vi "Utility_Read_Mixture_Cluster.vi"(6 "error in (no error)":errorcluster, 8 "Dir containing fluid files":path, 9 "Mixture File":path) -> (0 "error out":errorcluster, 3 "Mixure Cluster":T1)   [LabVIEW 2015]
doc: "Reads the .mix file from the disk and retruns a cluster specifying the composition of the fluid.\n\nDeveloped by:\nGreg Sussman\nProcess Automation Corp\nwww.processauto.com\n(267)685-1249"
uses:
  Ctl/Mixture Composition cluster_d.ctl
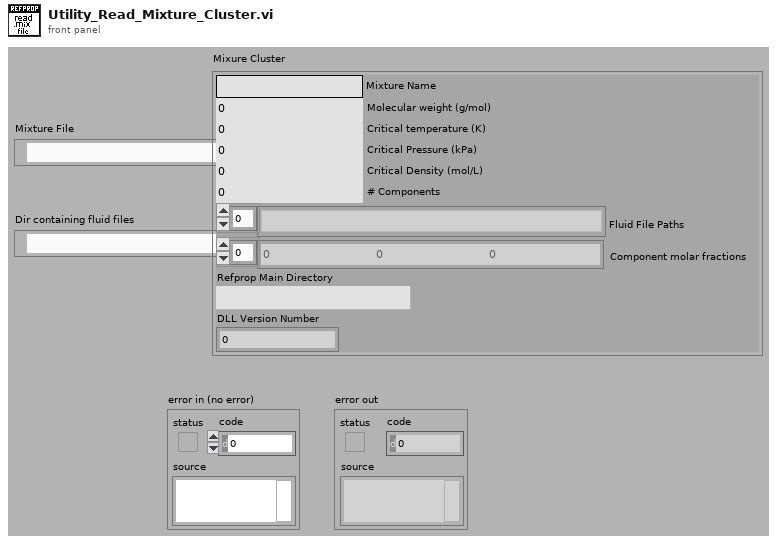
[diagram p1: front panel]
types:
  T1 = typedef "Mixture Composition cluster_d.ctl" = cluster{"Mixture Name":string, "Molecular weight (g/mol)":dbl, "Critical temperature (K)":dbl, "Critical Pressure (kPa)":dbl, "Critical Density (mol/L)":dbl, "# Components":i32, "Fluid File Paths":path[], "Component molar fractions":dbl[], "Refprop Main Directory":path, "DLL Version Number":dbl}
  T2 = enum16{"open", "open or create", "create or replace", "create", "open (read only)"}
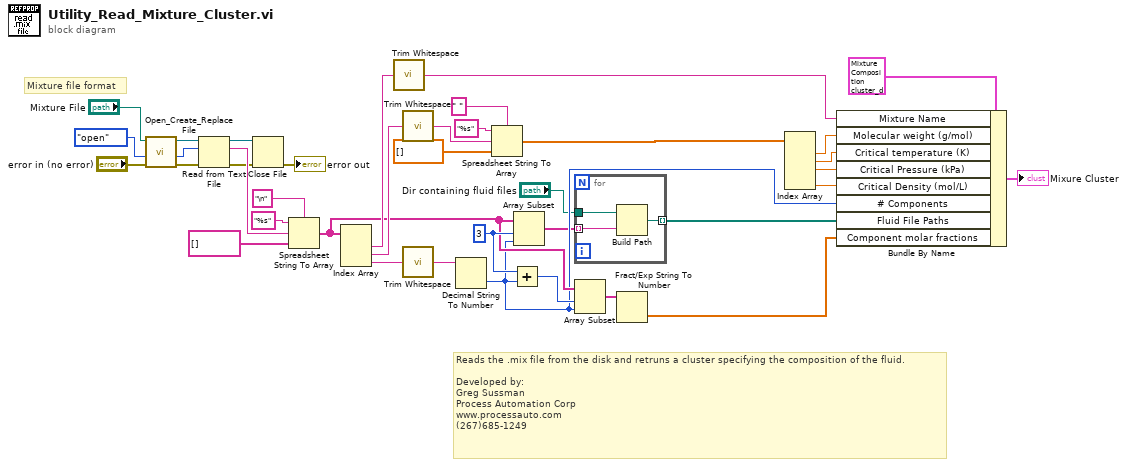
[diagram p0: block diagram]
diagram:
  w34 = 3 ("index")
  # "Reads the .mix file from the disk and retruns a cluster specifying the composition of the fluid.\n\nDeveloped by:\nGreg Sussman\nProcess Automation Corp\nwww.processauto.com\n(267)685-1249"
  # "Mixture file format"
  n1 = call <vilib>:"Open_Create_Replace File.vi"("error in (no error)"="error in (no error)", "function (open:0)"=T2."open", "file path"="Mixture File") -> ("error out"=w5:errorcluster, "file size (bytes)"=w1:i32, "refnum"=w4:refnum<file>)  [unwired: 5 in, 1 out]
  n2 = Read from Text File(file (use dialog)=w4, count=w1, error in=w5) -> (refnum out=w2:refnum<file>, text=w10:string, error out=w3:errorcluster)  [unwired: 1 in, 1 out]
  n3 = Close File(refnum=w2, error in=w3) -> (error out=→"error out":errorcluster)  [unwired: 1 out]
  n4 = Spreadsheet String To Array(delimiter (Tab)="\n", format string="%s", spreadsheet string=w10, array type (2D Dbl)=string[] []) -> (array=w18:string[])
  n5 = Index Array(array=w18) -> (element #1=w31:string, element #2=w24:string, element #3=w19:string)  [unwired: 3 in]
  n6 = call <vilib>:"Trim Whitespace.vi"("string"=w31) -> ("trimmed string"=w25:string)  [unwired: 1 in]
  n7 = call <vilib>:"Trim Whitespace.vi"("string"=w24) -> ("trimmed string"=w30:string)  [unwired: 1 in]
  n8 = call <vilib>:"Trim Whitespace.vi"("string"=w19) -> ("trimmed string"=w35:string)  [unwired: 1 in]
  n9 = Decimal String To Number(string=w35) -> (number=w17:i32)  [unwired: 2 in, 1 out]
  n10 = Spreadsheet String To Array(delimiter (Tab)=" ", format string="%s", spreadsheet string=w30, array type (2D Dbl)=dbl[] []) -> (array=w29:dbl[])
  n11 = Add(x=w34, y=w17) -> (x+y=w33:i32)
  n12 = Array Subset(array=w18, index=w34, length=w17) -> (w13:string[])
  n13 = for {
    tunnel: w13 -> [w41] mode=indexing
    tunnel: "Dir containing fluid files" -> [w40]
    tunnel: [w39] -> w11 mode=indexing
    n14 = Build Path(base path=w40, name or relative path=w41) -> (appended path=w39:path)
  }
  n15 = Array Subset(array=w18, index=w33, length=w17) -> (w32:string[])
  n16 = Fract/Exp String To Number(string=w32) -> (number=w15:dbl[])  [unwired: 3 in, 1 out]
  n17 = Index Array(array=w29) -> (element #1=w23:dbl, element #2=w22:dbl, element #3=w21:dbl, element #5=w20:dbl)  [unwired: 5 in, 1 out]
  n18 = Bundle By Name(cluster=T1 {"Mixture Name"="", "Molecular weight (g/mol)"=0.0, "Critical temperature (K)"=0.0, "Critical Pressure (kPa)"=0.0, "Critical Density (mol/L)"=0.0, "# Components"=0, "Fluid File Paths"=[], "Component molar fractions"=[], "Refprop Main Directory"=path "", "DLL Version Number"=0.0} ("Mixure Cluster"), "Mixture Name"=w25, "Molecular weight (g/mol)"=w23, "Critical temperature (K)"=w22, "Critical Pressure (kPa)"=w21, "Critical Density (mol/L)"=w20, "# Components"=w17, "Fluid File Paths"=w11, "Component molar fractions"=w15) -> (→"Mixure Cluster":T1)
